vi "簇波形图.vi"() -> ()   [LabVIEW 2018]
panel:
  out "波形图":waveform(dbl)(graph)
  out "波形输出":waveform(dbl)
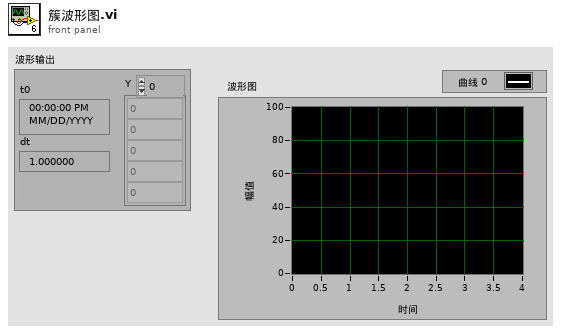
[diagram p1: front panel]
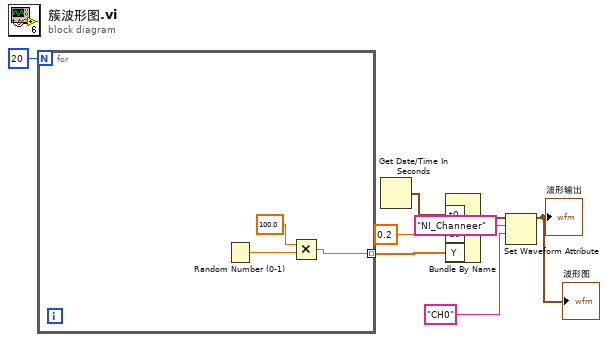
[diagram p0: block diagram]
diagram:
  n1 = for {
    N: 20 -> [_]
    tunnel: [w9] -> w7 mode=indexing
    n2 = Random Number (0-1)() -> (number: 0 to 1=w11:dbl)
    n3 = Multiply(x=100.0, y=w11) -> (x*y=w9:dbl)
  }
  n4 = Get Date/Time In Seconds() -> (seconds since 1Jan1904=w5:timestamp)
  n5 = Bundle By Name("t0"=w5, "dt"=0.2, "Y"=w7) -> (w4:waveform(dbl))  [unwired: 1 in]
  n6 = Set Waveform Attribute(5:"CH0", 6:"NI_Channeer" ("名称"), 7:w4) -> (3:→"波形输出" →"波形图":waveform(dbl))  [unwired: 1 in, 2 out]
